vi "build pulse idxes.vi"(9 "Output Valid":bool, 10 "rising edge!":bool, 11 "pulse idx in":u8) -> (2 "Numeric":u32, 3 "Boolean":bool)   [LabVIEW 2018, in "trigger-out.lvlib"]
uses:
  trigger-out.lvlib
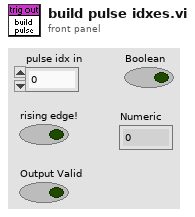
[diagram p1: front panel]
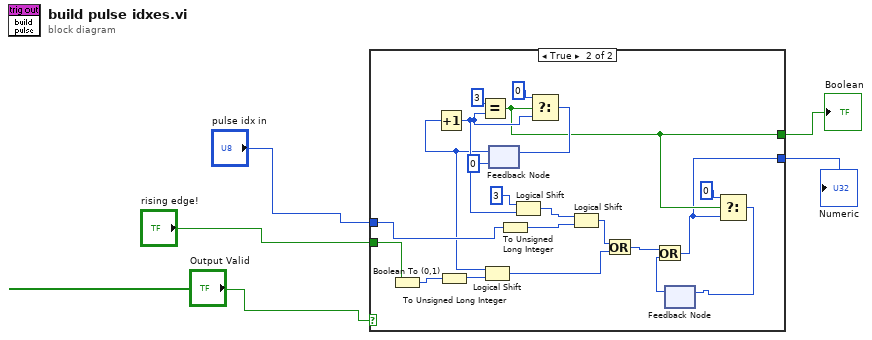
[diagram p0: block diagram]
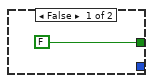
[diagram p2: hidden frame]
diagram:
  n1 = case shown="True" "Output Valid" {
    tunnel: [FALSE w10] -> w4
    tunnel: "rising edge!" -> [_ w19]
    tunnel: "pulse idx in" -> [_ w25]
    tunnel: [_ w8] -> w5
    frame False {
    }
    frame True {
      n2 = Boolean To (0,1)(Boolean=w19) -> (0, 1=w18:i16)
      n3 = To Unsigned Long Integer(number=w18) -> (unsigned 32bit integer=w17:u32)
      n4 = feedback #1(i16 0) -> (w16:i16)
      n5 = Increment(x=w16) -> (x+1=w22:i16)
      n6 = Equal?(x=i16 3, y=w22) -> (x = y?=w10:bool)
      n7 = Logical Shift(y=w16, x=w17) -> (x << y=w14:u32)
      n8 = To Unsigned Long Integer(number=w25) -> (unsigned 32bit integer=w23:u32)
      n9 = Logical Shift(y=i16 3, x=w22) -> (x << y=w20:i16)
      n10 = Select(t=i16 0, s=w10, f=w22) -> (s? t:f=w26:i16)
      n11 = feedback-in #1(w26) -> ()
      n12 = Logical Shift(y=w20, x=w23) -> (x << y=w15:u32)
      n13 = Or(x=w15, y=w14) -> (x .or. y?=w13:u32)
      n14 = feedback #2() -> (w12:u32)  [unwired: 1 in]
      n15 = Or(x=w13, y=w12) -> (x .or. y?=w8:u32)
      n16 = Select(t=i16 0, s=w10, f=w8) -> (s? t:f=w9:u32)
      n17 = feedback-in #2(w9) -> ()
    }
  }
  "Numeric" <- w5
  "Boolean" <- w4
